vi "acq.Image.vi"(7 "DVR":T2, 8 "error in":errorcluster) -> (0 "error out":errorcluster, 2 "Image Out":T1, 3 "buffer":u16[][](array[numeric]))   [LabVIEW 2020]
uses:
  _controls/data.ctl
  camera/camera.lvclass
  _controls/data.ref.ctl
  <vilib>/vision/Image Controls.llb/IMAQ Image.ctl
  _controls/state.ctl
  _controls/data.vars.ctl
  _controls/save_options.ctl
  _controls/flip.ctl
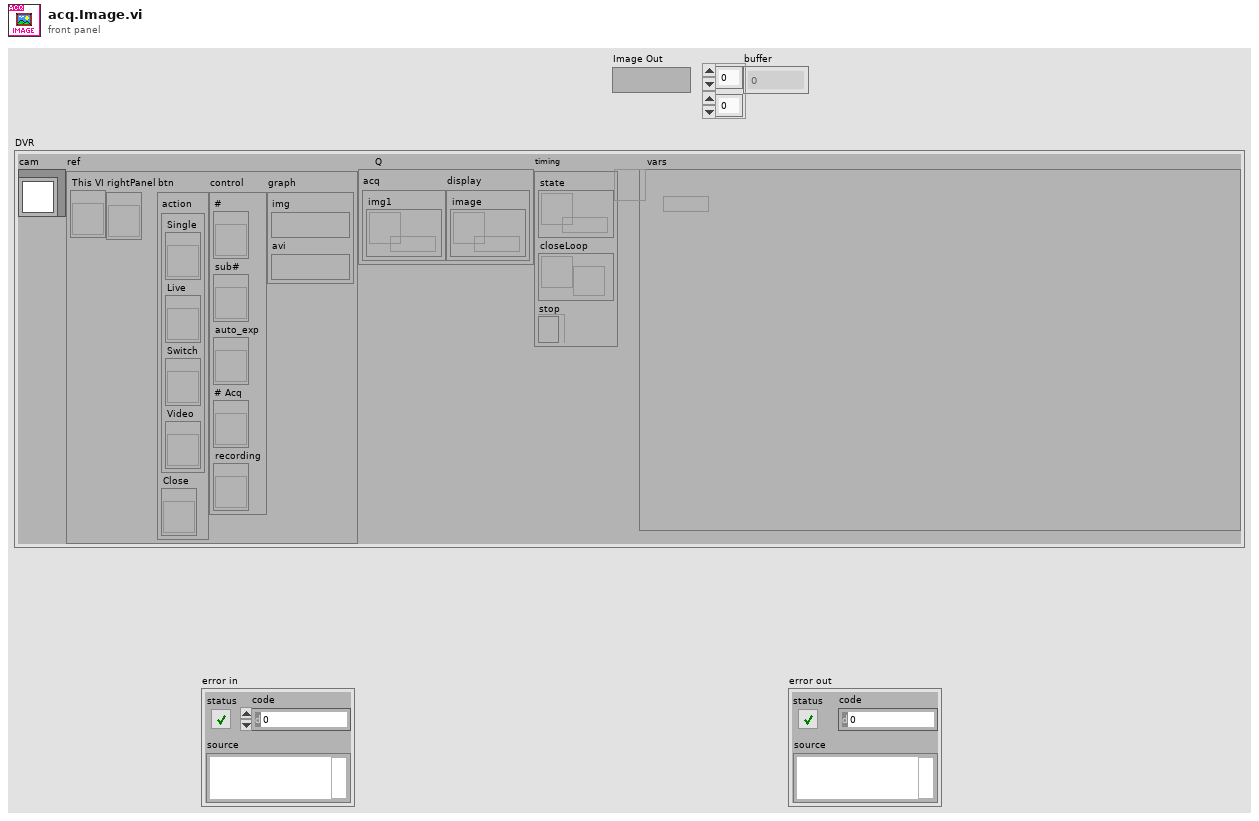
[diagram p1: front panel]
types:
  T1 = typedef "IMAQ Image.ctl" = refnum<image>
  T2 = typedef "data.ctl" = cluster{"cam":refnum<class "camera.lvclass">, "ref":T3, "Q":cluster{"acq":cluster{"img1":refnum<queue>}, "display":cluster{"image":refnum<queue>}}, "timing":cluster{"state":refnum<queue>, "closeLoop":refnum<notifier>, "stop":refnum<k4>}, "vars":refnum<data-value>}
  T3 = typedef "data.ref.ctl" = cluster{"This VI":refnum<vi>, "rightPanel":refnum<vi>, "btn":cluster{"action":cluster{"Single":refnum<vi>, "Live":refnum<vi>, "Switch":refnum<vi>, "Video":refnum<vi>}, "Close":refnum<vi>}, "control":cluster{"#":refnum<vi>, "sub#":refnum<vi>, "auto_exp":refnum<vi>, "# Acq":refnum<vi>, "recording":refnum<vi>}, "graph":cluster{"img":T1, "avi":T1}}
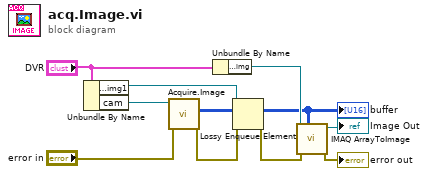
[diagram p0: block diagram]
diagram:
  n1 = Unbundle By Name("DVR") -> ("Q.acq.img1"=w5:refnum<queue>, "cam"=w7:refnum<class "camera.lvclass">)
  n2 = call-dynamic "Acquire.Image.vi"("error in"="error in", "camera.nit in"=w7) -> ("error out"=w2:errorcluster, "buffer"=w4:u16[][])  [unwired: 8 in]
  "buffer" <- w4
  n3 = Unbundle By Name("DVR") -> ("ref.graph.img"=w8:T1)
  n4 = Lossy Enqueue Element(queue=w5, element=w4, error in (no error)=w2) -> (error out=w3:errorcluster)  [unwired: 3 out]
  n5 = call "IMAQ ArrayToImage"("Image Pixels (U16)"=w4, "error in (no error)"=w3, "Image"=w8) -> ("error out"=→"error out":errorcluster, "Image Out"=→"Image Out":T1)  [unwired: 7 in]
